vi "WSVCAP SHL FPGA LL RFFE Write Data.vi"(0 "Bit In":bool, 11 "error in (no error)":errorcluster, 13 "Line":T1) -> (15 "error out":errorcluster)   [LabVIEW 2017]
uses:
  Type Defs/WSVCAP SHL RFFE Write Line Enum.ctl
  WSVCAP SHL FPGA LL RFFE Debug Global.vi
  <vilib>/eio/EIONode/EIONode.xnode
  <vilib>/rvi/eio/common/nirviEmuTemplateMethod_errors.vi
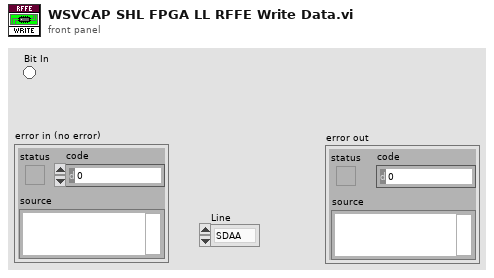
[diagram p1: front panel]
types:
  T1 = typedef "WSVCAP SHL RFFE Write Line Enum.ctl" = enum16{"SDAA", "SCLK"}
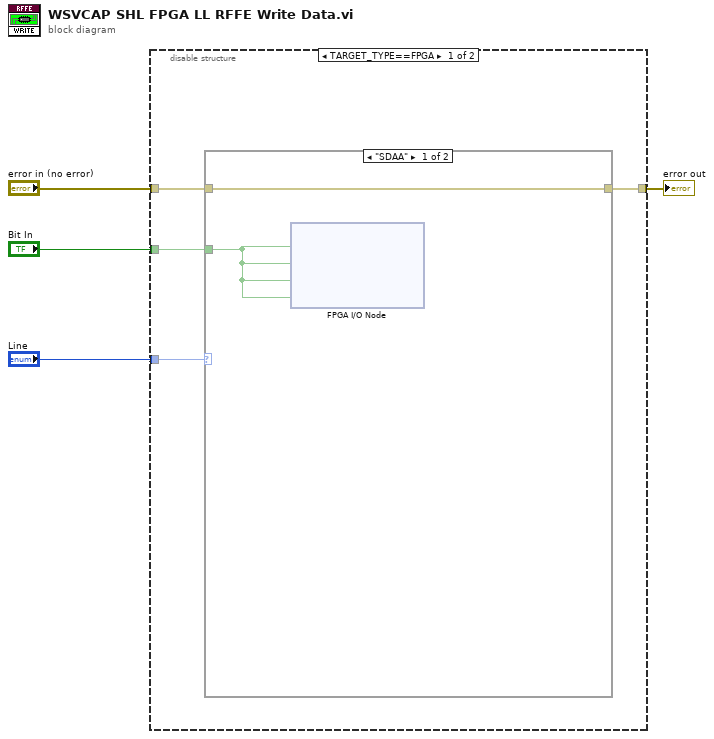
[diagram p0: block diagram]
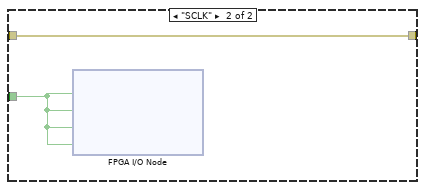
[diagram p2: hidden frame]
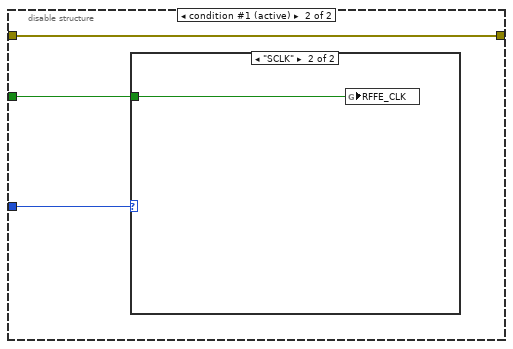
[diagram p3: hidden frame]
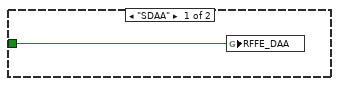
[diagram p4: hidden frame]
diagram:
  n1 = disable-structure shown="TARGET_TYPE==FPGA" {
    disable-tunnel: "Line" -> [w8 w15]
    disable-tunnel: [w7 w14] -> w3
    disable-tunnel: "error in (no error)" -> [w6 w14]
    disable-tunnel: "Bit In" -> [w5 w13]
    frame condition #0 {
      n2 = case shown="\"SDAA\"" w8 {
        tunnel: [w10 w12] -> w7
        tunnel: w6 -> [w10 w12]
        tunnel: w5 -> [w9 w11]
        frame "SDAA" {
          n3 = xnode "FPGA I/O Node"("RFFE_SDA_S1-16"=w9, "RFFE_SDA_S17-32"=w9, "RFFE_SDA_S33-48"=w9, "RFFE_SDA_S49-64"=w9) -> ()  [unwired: 4 in, 4 out]
        }
        frame "SCLK" {
          n4 = xnode "FPGA I/O Node"("RFFE_SCL_S1-16"=w11, "RFFE_SCL_S17-32"=w11, "RFFE_SCL_S33-48"=w11, "RFFE_SCL_S49-64"=w11) -> ()  [unwired: 4 in, 4 out]
        }
      }
    }
    frame condition #1 (active) {
      n5 = case shown="\"SCLK\"" w15 {
        tunnel: w13 -> [w16 w17]
        frame "SDAA" {
          n6 = global write "WSVCAP SHL FPGA LL RFFE Debug Global.vi" "RFFE_DAA"(w16) -> ()
        }
        frame "SCLK" {
          n7 = global write "WSVCAP SHL FPGA LL RFFE Debug Global.vi" "RFFE_CLK"(w17) -> ()
        }
      }
    }
  }
  "error out" <- w3
